vi "Lvi Write U32Data2D.vi"(0 "NumSamples":u32, 1 "NumChan":u32, 5 "TaskRef":i32, 7 "timeout":dbl, 9 "DataBuf":u32[](array[numeric])=array[4097 elements], 11 "error in (no error)":errorcluster, 12 "StartWrite":bool) -> (4 "NumQueued":u32, 6 "TaskRef out":i32, 8 "function return":i32, 15 "error out":errorcluster)   [LabVIEW 2022 SP3, in "DtLvLink.lvlib"]
doc: "Calls directly into the entry points of the DLL of the Data Acq SDK to write a data point from the specified task as a one-dimensional array of unsigned, 32-bit integers."
uses:
  DtLvLink.lvlib
  <userlib>/LV-Link3/DtLvLink_64.dll
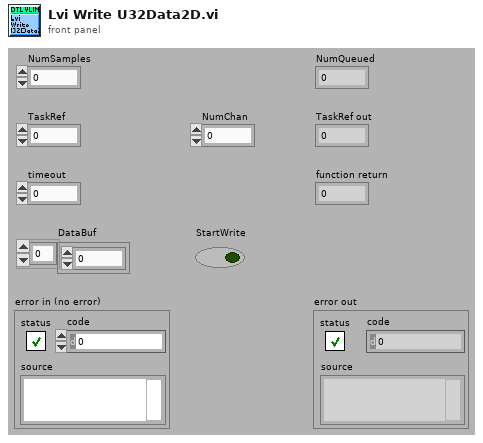
[diagram p1: front panel]
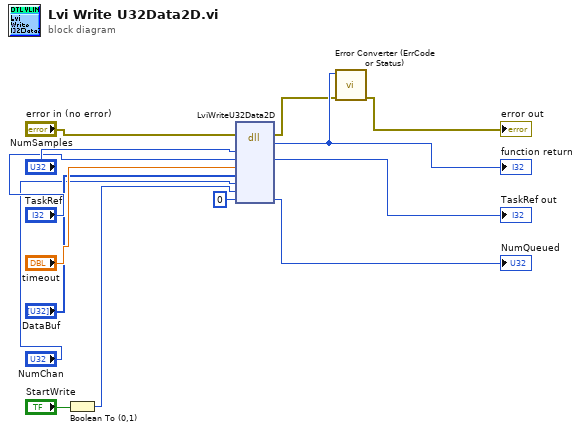
[diagram p0: block diagram]
diagram:
  n1 = Boolean To (0,1)(Boolean="StartWrite") -> (0, 1=w6:i16)
  n2 = dll-call lib="C:/Program Files/National Instruments/LabVIEW 2022/user.lib/LV-Link3/DtLvLink_64.*" fn="LviWriteU32Data2D"(error in="error in (no error)", "NumSamples"="NumSamples", "TaskRef"="TaskRef", "timeout"="timeout", "DataBuf"="DataBuf", "NumChan"="NumChan", "StartWrite"=w6, "NumQueued"=u32 0) -> (error out=w2:errorcluster, "return type"=w14:i32, "TaskRef"=→"TaskRef out":i32, "NumQueued"=→"NumQueued":u32)  [unwired: 7 in, 1 out]
  "function return" <- w14
  n3 = call "Error Converter (ErrCode or Status).vi"("error in (no error)"=w2, "error code"=w14) -> ("error out"=→"error out":errorcluster)  [unwired: 9 in]
